vi "Get SMO Port.vi"(8 "error in (no error)":errorcluster, 11 "Inst.SPCInstrument in":refnum<class "Inst.SPC.lvclass">) -> (0 "error out":errorcluster, 2 "Port":u16, 3 "Inst.SPCInstrument out":refnum<class "Inst.SPC.lvclass">)   [LabVIEW 2019, in "Inst.SPC.lvclass"]
uses:
  Inst.SPC.lvclass
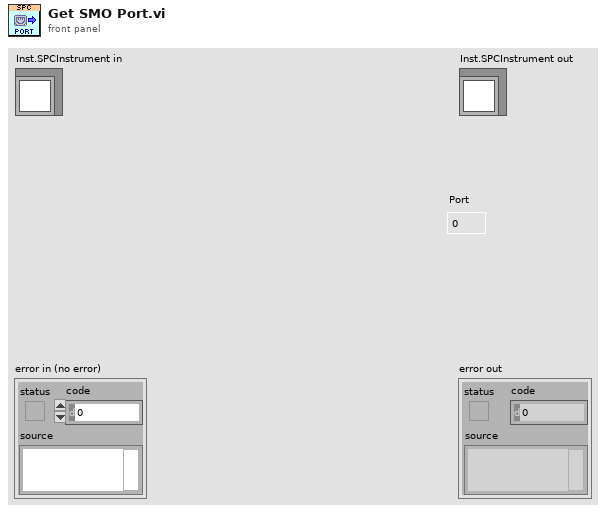
[diagram p1: front panel]
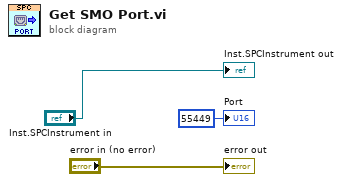
[diagram p0: block diagram]
diagram:
  "error out" <- "error in (no error)"
  "Inst.SPCInstrument out" <- "Inst.SPCInstrument in"
  "Port" <- u16 55449 ("Port")
